vi "com.vi"(7 "VISA resource name":refnum<visa-resource-name>="COM1", 8 "stop":bool, 9 "Write String":string, 10 "Write":bool, 11 "baud rate (9600)":u32=9600) -> (1 "Read String":string)   [LabVIEW 2010]
uses:
  <vilib>/Instr/_visa.llb/VISA Configure Serial Port (Instr).vi
panel:
  in  "数据长度":u16
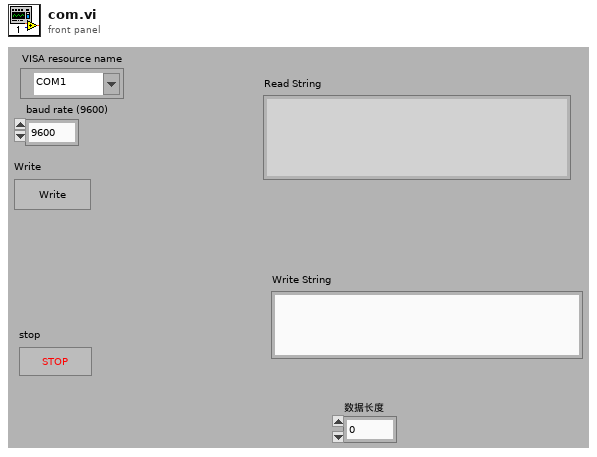
[diagram p1: front panel]
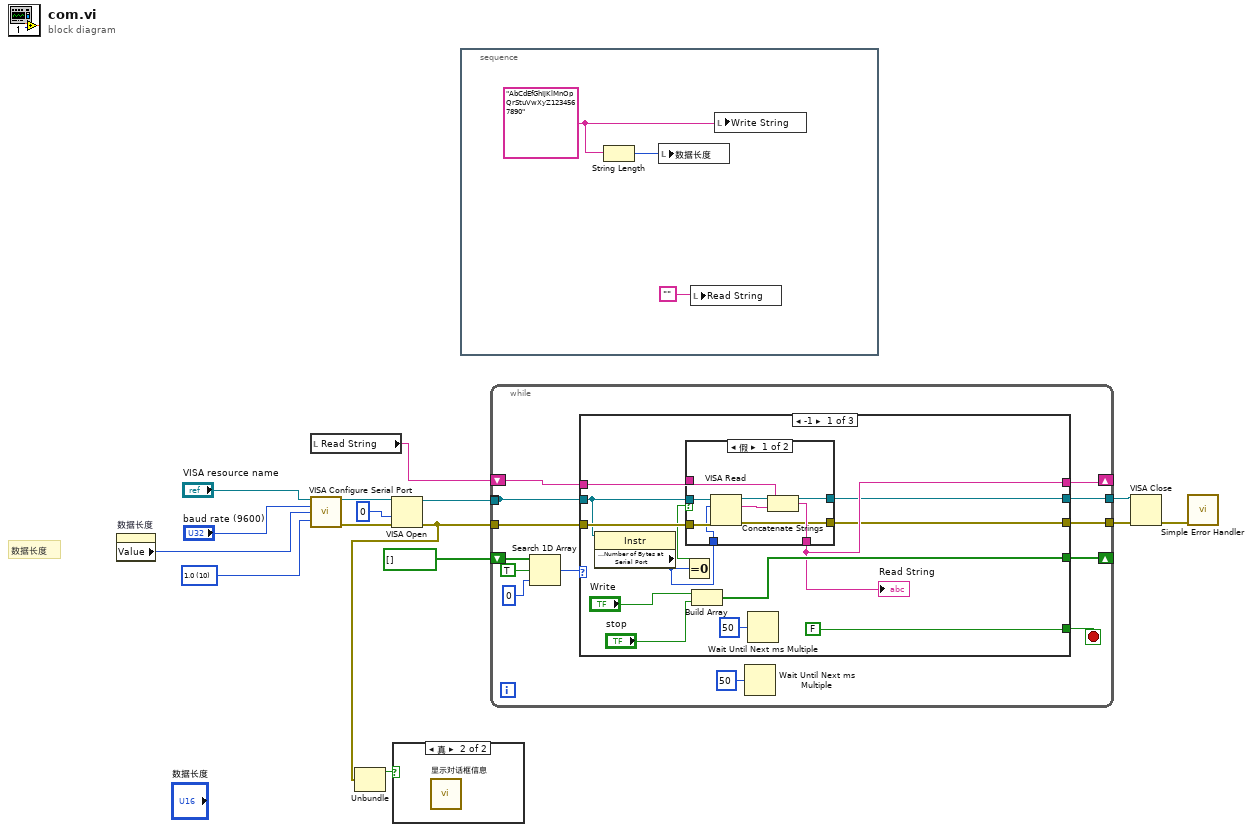
[diagram p0: block diagram]
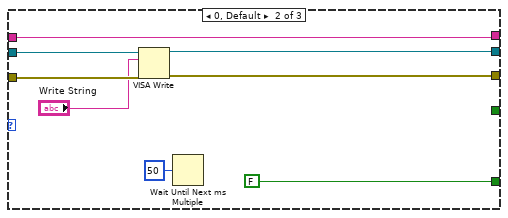
[diagram p4: hidden frame]
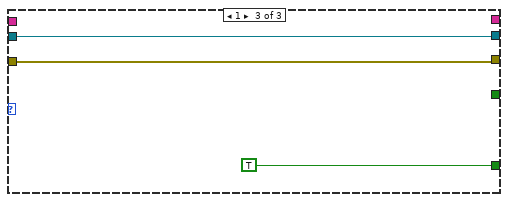
[diagram p5: hidden frame]
diagram:
  w4 = u16 10 items=["1.0"=10, "1.5"=15, "2.0"=20] ("stop bits (10: 1 bit)")
  # "数据长度"
  n1 = property on="数据长度" class="DigNum (严格)"() -> ("Value"=w1:u16)  [unwired: 2 in, 2 out]
  n2 = local read "Read String"() -> (w2:string)
  n3 = call-poly "VISA Configure Serial Port"("VISA resource name"="VISA resource name", "baud rate (9600)"="baud rate (9600)", "data bits (8)"=w1, "stop bits (10: 1 bit)"=w4) -> ("VISA resource name out"=w10:refnum<visa-resource-name>, "error out"=w6:errorcluster)  [unwired: 10 in]
  n4 = VISA Open(access mode=u32 0, error in (no error)=w6, VISA resource name=w10) -> (VISA resource name=w9:refnum<visa-resource-name>, error out=w3:errorcluster)  [unwired: 2 in]
  n5 = Unbundle(w3) -> ("status"=w5:bool)  [unwired: 2 out]
  n6 = case shown="真" w5 {
    frame False {
    }
    frame True {
      n7 = call "显示对话框信息"() -> ()  [unwired: 10 in, 2 out]
    }
  }
  n8 = stacked-sequence {
    frame #0 {
      w17 = "AbCdEfGhIjKlMnOpQrStuVwXyZ1234567890"
      n9 = String Length(string=w17) -> (length=w16:i32)
      n10 = local write "数据长度"(w16) -> ()
      n11 = local write "Read String"("") -> ()
      n12 = local write "Write String"(w17) -> ()
    }
  }
  n13 = while {
    tunnel: [w20] -> _
    shift-right: [w27] -> _
    shift-left: bool[] [] -> [w31]
    tunnel: w3 -> [w26]
    shift-right: [w24] -> _
    shift-left: w2 -> [w25]
    tunnel: [w23] -> w13
    tunnel: [w22] -> w12
    tunnel: w9 -> [w20]
    stop <- w21 stop-if-true
    n14 = Search 1D Array(1D array=w31, element=TRUE, start index (0)=0) -> (index of element=w28:i32)
    n15 = case shown="-1" w28 {
      tunnel: [w42 _ _] -> w27
      tunnel: w20 -> [w35 w63 w65]
      tunnel: w26 -> [w41 w62 w64]
      tunnel: w25 -> [w39 w59 _]
      tunnel: [w40 w59 _] -> w24
      tunnel: [w38 w61 w65] -> w23
      tunnel: [w37 w60 w64] -> w22
      tunnel: [FALSE FALSE TRUE] -> w21
      frame -1 {
        n16 = property class="Instr"(reference=w35) -> ("Serial Settings:Number of Bytes at Serial Port"=w32:u32)  [unwired: 1 in, 2 out]
        n17 = Equal To 0?(x=w32) -> (x = 0?=w33:bool)
        n18 = case shown="假" w33 {
          tunnel: w41 -> [w52 w54]
          tunnel: [w51 w53] -> w40
          tunnel: w39 -> [w50 w53]
          tunnel: [w48 w55] -> w38
          tunnel: [w47 w54] -> w37
          tunnel: w35 -> [w46 w55]
          tunnel: w32 -> [w45 _]
          frame False {
            n19 = VISA Read(VISA resource name=w46, byte count=w45, error in (no error)=w52) -> (VISA resource name out=w48:refnum<visa-resource-name>, read buffer=w49:string, error out=w47:errorcluster)  [unwired: 1 out]
            n20 = Concatenate Strings(w50, w49) -> (w51:string)
          }
          frame True {
          }
        }
        "Read String" <- w40
        n21 = Build Array("Write", "stop") -> (w42:bool[])
        n22 = Wait Until Next ms Multiple(millisecond multiple=u32 50 ("milliseconds to wait")) -> ()  [unwired: 1 out]
      }
      frame 0, Default {
        n23 = VISA Write(VISA resource name=w63, write buffer="Write String", error in (no error)=w62) -> (VISA resource name out=w61:refnum<visa-resource-name>, error out=w60:errorcluster)  [unwired: 1 out]
        n24 = Wait Until Next ms Multiple(millisecond multiple=u32 50 ("milliseconds to wait")) -> ()  [unwired: 1 out]
      }
      frame 1 {
      }
    }
    n25 = Wait Until Next ms Multiple(millisecond multiple=u32 50 ("milliseconds to wait")) -> ()  [unwired: 1 out]
  }
  n26 = VISA Close(VISA resource name=w13, error in (no error)=w12) -> (error out=w11:errorcluster)
  n27 = call <vilib>:"Simple Error Handler.vi"("error in (no error)"=w11) -> ()  [unwired: 4 in, 5 out]
